vi "Master - Add EtherCAT Slave.vi"(8 "error in (no error)":errorcluster, 11 "Node Ptr":u64 format="%.0x") -> (0 "error out":errorcluster)   [LabVIEW 2019, in "Scan Engine Custom Device.lvlib"]
uses:
  Scan Engine Custom Device.lvlib
  Type Defs/NI ECAT Slaves.ctl
  Globals/Scan Engine GUIDs.vi
  Globals/Property Strings.vi
  <vilib>/NI VeriStand/Custom Device API/Custom Device API.lvlib
panel:
  in  "Tag":string
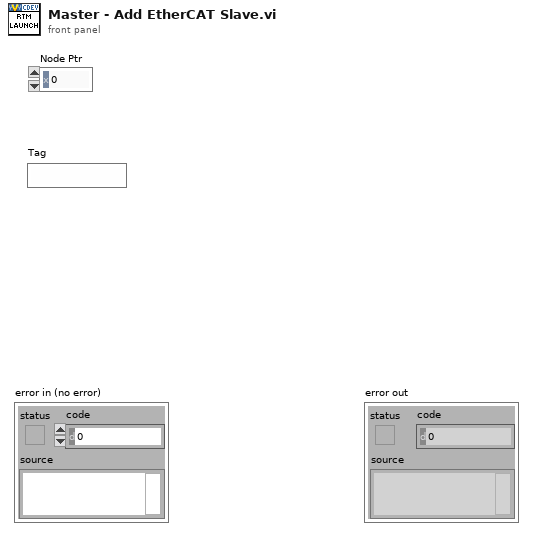
[diagram p1: front panel]
types:
  T1 = typedef "Scan Engine Custom Device.lvlib/NI ECAT Slaves.ctl" = enum16{"Default", "NI 9144"}
  T2 = typedef "Custom Device API.lvlib/Custom Device Item Ref.ctl" = u64
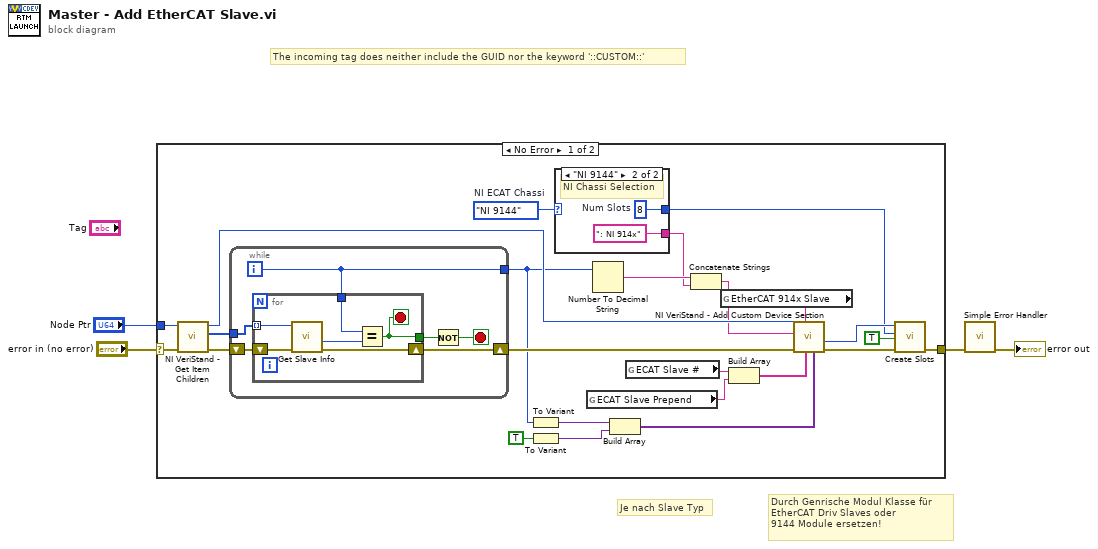
[diagram p0: block diagram]
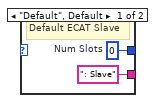
[diagram p2: hidden frame]
diagram:
  # "Durch Genrische Modul Klasse für \nEtherCAT Driv Slaves oder \n9144 Module ersetzen!"
  # "Je nach Slave Typ"
  # "The incoming tag does neither include the GUID nor the keyword '::CUSTOM::'"
  n1 = case shown="No Error" "error in (no error)" {
    selector: "error in (no error)" -> [w15 w45]
    tunnel: "Node Ptr" -> [w16 _]
    tunnel: [w14 w45] -> w2
    frame No Error {
      w7 = NI_ECAT_Slaves."NI 9144"  # NI ECAT Chassi
      n2 = call <vilib>:"NI VeriStand - Get Item Children.vi"("error in (no error)"=w15, "Item Ref in"=w16) -> ("error out"=w28:errorcluster, "Child Refs"=w27:T2[], "Item Ref out"=w24:T2)  [unwired: 6 in, 1 out]
      n3 = while {
        shift-right: [w34] -> w25
        shift-left: w28 -> [w38]
        tunnel: w27 -> [w37]
        tunnel: [w33] -> w9
        i -> [w33]
        stop <- w35 stop-if-true
        n4 = for {
          tunnel: w37 -> [w41] mode=indexing
          shift-right: [w40] -> w34
          shift-left: w38 -> [w42]
          tunnel: w33 -> [w44]
          tunnel: [w43] -> w36
          stop <- w43 stop-if-true
          n5 = call "Get Slave Info.vi"("error in (no error)"=w42, "Item Ref in"=w41) -> ("error out"=w40:errorcluster, "Slave #"=w39:u16)  [unwired: 5 in, 3 out]
          n6 = Equal?(x=w44, y=w39) -> (x = y?=w43:bool)
        }
        n7 = Not(x=w36) -> (.not. x?=w35:bool)
      }
      n8 = To Variant(anything=w9) -> (Variant=w10:variant)
      n9 = To Variant(anything=TRUE) -> (Variant=w11:variant)
      n10 = case "Case-Struktur" shown="\"NI 9144\"" w7 {
        tunnel: [w30 w32] -> w6
        tunnel: [": Slave" ("string") ": NI 914x" ("string")] -> w5
        frame "Default", Default {
          w30 = 0  # Num Slots
          # "Default ECAT Slave"
        }
        frame "NI 9144" {
          w32 = 8  # Num Slots
          # "NI Chassi Selection"
        }
      }
      n11 = global read "Property Strings.vi" "ECAT Slave Prepend"() -> (w13:string)
      n12 = Number To Decimal String(number=w9) -> (decimal integer string=w21:string)  [unwired: 1 in]
      n13 = Build Array(w10, w11) -> (w8:variant[])
      n14 = global read "Property Strings.vi" "ECAT Slave #"() -> (w23:string)
      n15 = Concatenate Strings(w21, w5) -> (w20:string)
      n16 = global read "Scan Engine GUIDs.vi" "EtherCAT 914x Slave"() -> (w26:string)
      n17 = Build Array(w23, w13) -> (w22:string[])
      n18 = call <vilib>:"NI VeriStand - Add Custom Device Section.vi"("Property Values"=w8, "Property names"=w22, "GUID (Default Section)"=w26, "error in (no error)"=w25, "Section Name"=w20, "Parent Ref in"=w24) -> ("error out"=w18:errorcluster, "Section Ptr"=w17:T2)  [unwired: 2 in, 2 out]
      n19 = call "Create Slots.vi"("error in"=w18, "EtherCAT?"=TRUE, "Num Slots"=w6, "Item Ref In"=w17) -> ("error out"=w14:errorcluster)  [unwired: 3 in, 3 out]
    }
    frame Error {
    }
  }
  n20 = call <vilib>:"Simple Error Handler.vi"("error in (no error)"=w2) -> ("error out"=→"error out":errorcluster)  [unwired: 4 in, 4 out]
